vi "Get LocalAppData Base Path.vi"(8 "error in (no error)":errorcluster, 11 "Operating System":string) -> (0 "error out":errorcluster, 3 "Path":path)   [LabVIEW 2020, in "RxnRover.lvlib" / "File IO.lvlib"]
doc: "Uses command prompt based off of the current operating system to retrive the LocalAppData base path\nSupports: Windows 2000 - Windows 11, Linux, Mac OS\n\nCreated 5/20/2025 - Labview 2020\nRxnRover"
uses:
  File IO.lvlib
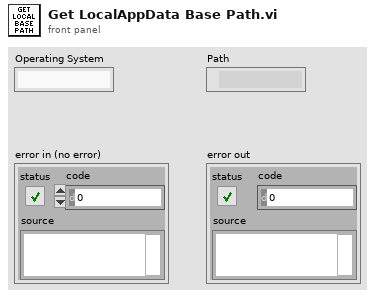
[diagram p1: front panel]
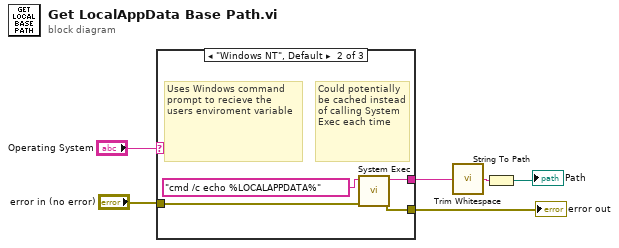
[diagram p0: block diagram]
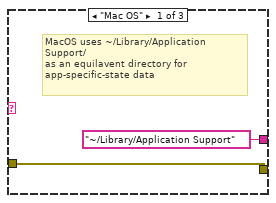
[diagram p2: hidden frame]
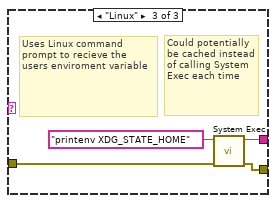
[diagram p3: hidden frame]
diagram:
  n1 = case shown="\"Windows NT\", Default" "Operating System" {
    tunnel: "error in (no error)" -> [w8 w12 w16]
    tunnel: [w8 w11 w14] -> w2
    tunnel: ["~/Library/Application Support" ("standard output") w10 w15] -> w5
    frame "Mac OS" {
      # "MacOS uses ~/Library/Application Support/ \nas an equilavent directory for app-specific-state data"
    }
    frame "Windows NT", Default {
      # "Could potentially be cached instead of calling System Exec each time"
      # "Uses Windows command prompt to recieve the users enviroment variable"
      n2 = call <vilib>:"System Exec.vi"("error in (no error)"=w12, "command line"="cmd /c echo %LOCALAPPDATA%" ("standard input")) -> ("error out"=w11:errorcluster, "standard output"=w10:string)  [unwired: 6 in, 2 out]
    }
    frame "Linux" {
      # "Could potentially be cached instead of calling System Exec each time"
      # "Uses Linux command prompt to recieve the users enviroment variable"
      n3 = call <vilib>:"System Exec.vi"("error in (no error)"=w16, "command line"="printenv XDG_STATE_HOME" ("standard input")) -> ("error out"=w14:errorcluster, "standard output"=w15:string)  [unwired: 6 in, 2 out]
    }
  }
  "error out" <- w2
  n4 = call <vilib>:"Trim Whitespace.vi"("string"=w5) -> ("trimmed string"=w4:string)  [unwired: 1 in]
  n5 = String To Path(string=w4) -> (path=→"Path":path)
